vi "sub vi - Log udate V2.vi"(10 "data":T1, 11 "panel id":string) -> (0 "error out":errorcluster)   [LabVIEW 2013]
uses:
  program files/Global 1.vi
  <vilib>/Utility/file.llb/Write To Spreadsheet File (string).vi
panel:
  in  "file dir":string
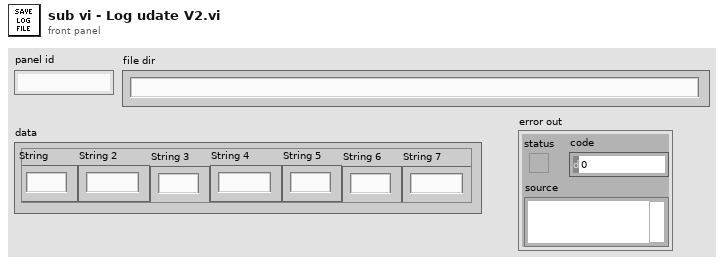
[diagram p1: front panel]
types:
  T1 = cluster{"String":string, "String 2":string, "String 3":string, "String 4":string, "String 5":string, "String 6":string, "String 7":string}
  T2 = enum16{"open", "replace", "create", "open or create", "replace or create", "replace or create with confirmation"}
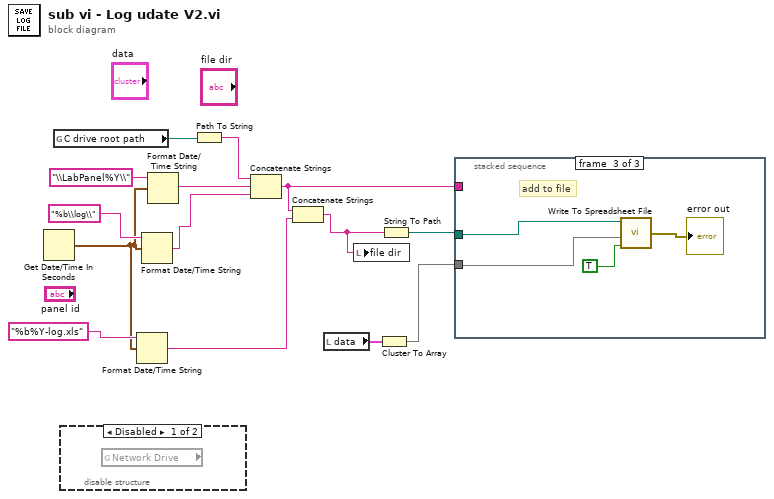
[diagram p0: block diagram]
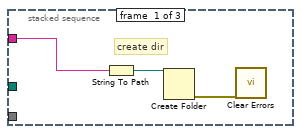
[diagram p2: hidden frame]
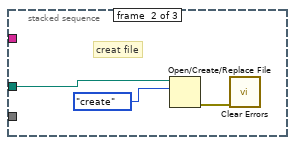
[diagram p3: hidden frame]
diagram:
  n1 = Get Date/Time In Seconds() -> (seconds since 1Jan1904=w7:timestamp)
  n2 = global read "Global 1.vi" "C drive root path"() -> (w12:path)
  n3 = disable-structure shown="Disabled" {
    frame Disabled {
      n4 = global read "Global 1.vi" "Network Drive"() -> ()  [unwired: 1 out]
    }
    frame Enabled {
    }
  }
  n5 = Format Date/Time String(time format string (%c)="%b%Y-log.xls", seconds (now)=w7) -> (date/time string=w1:string)  [unwired: 1 in]
  n6 = Format Date/Time String(time format string (%c)="%b\\log\\", seconds (now)=w7) -> (date/time string=w9:string)  [unwired: 1 in]
  n7 = Format Date/Time String(time format string (%c)="\\LabPanel%Y\\", seconds (now)=w7) -> (date/time string=w10:string)  [unwired: 1 in]
  n8 = Path To String(path=w12) -> (string=w11:string)
  n9 = Concatenate Strings(w11, w10, w9) -> (w5:string)
  n10 = Concatenate Strings(w5, w1) -> (w4:string)
  n11 = local read "data"() -> (w3:T1)
  n12 = local write "file dir"(w4) -> ()
  n13 = Cluster To Array(cluster=w3) -> (array=w2:string[])
  n14 = String To Path(string=w4) -> (path=w6:path)
  n15 = stacked-sequence {
    tunnel: w6 -> [_ w18 w23]
    tunnel: w2 -> [_ _ w22]
    tunnel: w5 -> [w16 _ _]
    frame #0 {
      # "create dir"
      n16 = String To Path(string=w16) -> (path=w17:path)
      n17 = Create Folder(path (use dialog)=w17) -> (error out=w15:errorcluster)  [unwired: 2 in, 2 out]
      n18 = call <vilib>:"Clear Errors.vi"("error in (no error)"=w15) -> ()  [unwired: 6 in, 1 out]
    }
    frame #1 {
      # "creat file"
      n19 = Open/Create/Replace File(file path (use dialog)=w18, operation (0:open)=T2."create") -> (error out=w19:errorcluster)  [unwired: 4 in, 2 out]
      n20 = call <vilib>:"Clear Errors.vi"("error in (no error)"=w19) -> ()  [unwired: 6 in, 1 out]
    }
    frame #2 {
      # "add to file"
      n21 = call-poly <vilib>:"Write To Spreadsheet File.vi"("append to file? (new file:F)"=TRUE, "1D data"=w22, "file path (dialog if empty)"=w23) -> ("error out"=→"error out":errorcluster)  [unwired: 4 in, 1 out]
    }
  }
